vi "PassFail.vi"(0 "Failed: 2":string, 1 "STATUS":bool) -> ()   [LabVIEW 2011]
panel:
  out "Failed:":string
  in  "OK Button":bool caption="PASS"
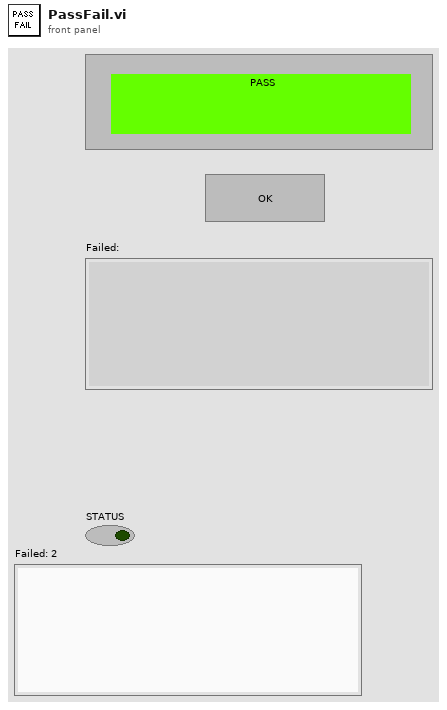
[diagram p1: front panel]
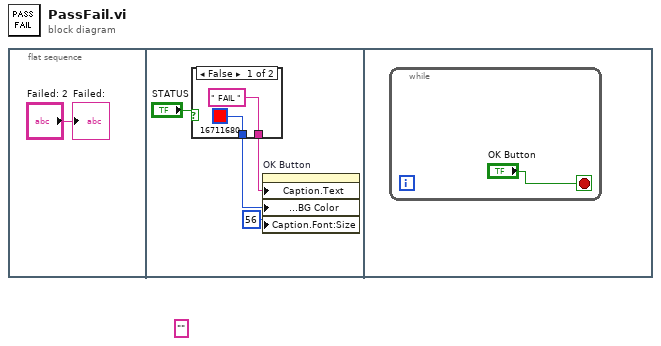
[diagram p0: block diagram]
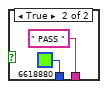
[diagram p2: hidden frame]
diagram:
  (unwired) "" ("String")
  n1 = flat-sequence {
    frame #0 {
      "Failed:" <- "Failed: 2"
    }
    frame #1 {
      n2 = case shown="False" "STATUS" {
        tunnel: [u32 16711680 ("Text.Colors:BG Color") u32 6618880 ("Text.Colors:BG Color")] -> w4
        tunnel: [" FAIL " ("Text.Text") " PASS " ("Text.Text")] -> w3
        frame False {
        }
        frame True {
        }
      }
      n3 = property on="OK Button" class="Bool"("Caption.Text"=w3, "Caption.Text Colors:BG Color"=w4, "Caption.Font:Size"=u32 56) -> ()  [unwired: 2 in, 2 out]
    }
    frame #2 {
      n4 = while {
        stop <- "OK Button" stop-if-true
      }
    }
  }
